vi "SVFA Compensate Phase for Ref Freq and Harm (Complex) (1 Ch).vi"(0 "complex spectrum":T7={"complex spectrum response"={"f0"=0.0, "df"=1.0, "complex spectrum"=[]}, "spectrum info"={"channel name"="", "description"="", "x-axis units"=0, "spectral info"={"spectrum type"=enum."Power [Magnitude^2]", "linear/dB"=enum."linear", "window"=0, "window size"=0, "FFT size"=0}, "engineering units"=0, "custom label"="", "dB reference [EU]"=0.0, "peak units"=enum."rms", "weighting filter"=0, "spectral density?"=FALSE, "unit label"="", "spectrum skewed?"=FALSE, "complimentary spectrum units"=enum."none"}} {"spectrum info"."x-axis units" items=["Time (s)"=0, "Frequency-CB (Hz)"=1, "Frequency-CPB (Hz)"=1248, "Frequency-Arbitrary (Hz)"=2357, "Quefrency (s)"=2, "Revolutions (rev)"=3, "Order"=4, "Speed (RPM)"=11, "Speed (rad/s)"=21, "Index"=65535]; "spectrum info"."weighting filter" items=["Linear", "A-weighting", "B-weighting", "C-weighting", "ITU-R 468-4", "Dolby", "CCITT", "C-message", "Wb", "Wc", "Wd", "We", "Wf", "Wh", "Wj", "Wk", "Wm", "AES17 20 kHz lowpass", "AES17 40 kHz lowpass", "AES17 20 kHz highpass", "AES17 40 kHz highpass"]; "spectrum info"."dB reference [EU]" format="%.2f"; "spectrum info"."engineering units" items=["custom..."=0, "V"=1, "A"=21, "C"=30, "pC"=31, "s"=32, "-"=29, "Pa"=2, "N"=20, "g"=3, "m/s^2"=4, "m/s"=5, "m"=6, "mm/s"=12, "mm"=13, "micron/s"=14, "micron"=15, "in/s^2"=7, "in/s"=8, "in"=9, "mil/s"=10, "mil"=11, "rad/s^2"=16, "rad/s"=17, "rad"=18, "deg/s^2"=26, "deg/s"=27, "deg"=28, "RPM"=22, "cycle/s^2"=23, "Hz"=24, "cycle"=25, "strain"=19]; "spectrum info"."spectral info"."window" items=["None "=0, "Hanning"=1, "Hamming"=2, "Blackman-Harris"=3, "Exact Blackman"=4, "Blackman"=5, "Flat Top"=6, "4 Term B-Harris "=7, "7 Term B-Harris"=8, "Low Sidelobe"=9, "Force - Exponential"=10, "Gaussian"=62]; "complex spectrum response"."complex spectrum" format="%.2f"; "complex spectrum response"."df" format="%.2f"; "complex spectrum response"."f0" format="%.2f"}, 2 "reference frequency [Hz]":dbl=-1.0, 3 "advanced span [Hz]":dbl, 5 "error in":errorcluster) -> (14 "phase compensated complex spectrum":T7={"complex spectrum response"={"f0"=0.0, "df"=1.0, "complex spectrum"=[]}, "spectrum info"={"channel name"="", "description"="", "x-axis units"=0, "spectral info"={"spectrum type"=enum."Power [Magnitude^2]", "linear/dB"=enum."linear", "window"=0, "window size"=0, "FFT size"=0}, "engineering units"=0, "custom label"="", "dB reference [EU]"=0.0, "peak units"=enum."rms", "weighting filter"=0, "spectral density?"=FALSE, "unit label"="", "spectrum skewed?"=FALSE, "complimentary spectrum units"=enum."none"}} {"spectrum info"."x-axis units" items=["Time (s)"=0, "Frequency-CB (Hz)"=1, "Frequency-CPB (Hz)"=1248, "Frequency-Arbitrary (Hz)"=2357, "Quefrency (s)"=2, "Revolutions (rev)"=3, "Order"=4, "Speed (RPM)"=11, "Speed (rad/s)"=21, "Index"=65535]; "spectrum info"."weighting filter" items=["Linear", "A-weighting", "B-weighting", "C-weighting", "ITU-R 468-4", "Dolby", "CCITT", "C-message", "Wb", "Wc", "Wd", "We", "Wf", "Wh", "Wj", "Wk", "Wm", "AES17 20 kHz lowpass", "AES17 40 kHz lowpass", "AES17 20 kHz highpass", "AES17 40 kHz highpass"]; "spectrum info"."dB reference [EU]" format="%.2f"; "spectrum info"."engineering units" items=["custom..."=0, "V"=1, "A"=21, "C"=30, "pC"=31, "s"=32, "-"=29, "Pa"=2, "N"=20, "g"=3, "m/s^2"=4, "m/s"=5, "m"=6, "mm/s"=12, "mm"=13, "micron/s"=14, "micron"=15, "in/s^2"=7, "in/s"=8, "in"=9, "mil/s"=10, "mil"=11, "rad/s^2"=16, "rad/s"=17, "rad"=18, "deg/s^2"=26, "deg/s"=27, "deg"=28, "RPM"=22, "cycle/s^2"=23, "Hz"=24, "cycle"=25, "strain"=19]; "spectrum info"."spectral info"."window" items=["None "=0, "Hanning"=1, "Hamming"=2, "Blackman-Harris"=3, "Exact Blackman"=4, "Blackman"=5, "Flat Top"=6, "4 Term B-Harris "=7, "7 Term B-Harris"=8, "Low Sidelobe"=9, "Force - Exponential"=10, "Gaussian"=62]; "complex spectrum response"."complex spectrum" format="%.2f"; "complex spectrum response"."df" format="%.2f"; "complex spectrum response"."f0" format="%.2f"}, 19 "error out":errorcluster)   [LabVIEW 2017]
doc: "Use this VI to enable vector averaging of complex spectra even when the frequencies of interest do not have constant phase incidence in the measurement window (analysis block)."
uses:
  <vilib>/addons/_NISVFA/_Shared subVIs/Controls/svc_Spectrum Info.ctl
  <vilib>/addons/_NISVFA/_Shared subVIs/Controls/svc_X-Axis Units.ctl
  <vilib>/addons/_NISVFA/_Shared subVIs/Controls/svc_Spectrum Type.ctl
  <vilib>/addons/_NISVFA/_Shared subVIs/Controls/svc_Engineering Units Text Ring.ctl
  <vilib>/addons/_NISVFA/_Shared subVIs/Controls/svc_Weighting Filter Text Ring.ctl
  <vilib>/addons/_NISVFA/_Shared subVIs/Controls/svc_Complimentary Spectrum Units.ctl
  <vilib>/addons/_NISVFA/_Spectrum Processing/SVFA Extract Single Tone Information (Complex) (1 Ch).vi
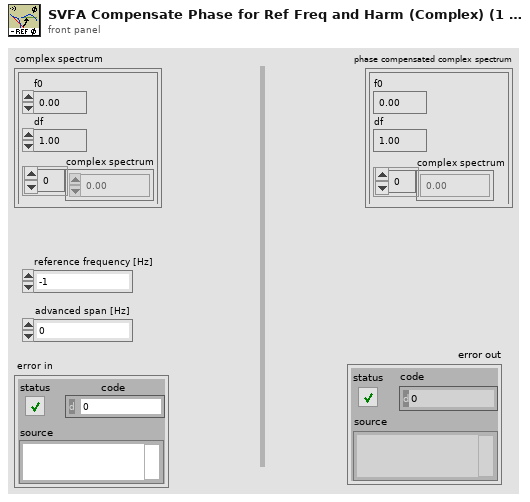
[diagram p1: front panel]
types:
  T1 = typedef "svc_Spectrum Info.ctl" = cluster{"channel name":string, "description":string, "x-axis units":T2, "spectral info":cluster{"spectrum type":T3, "linear/dB":enum16{"linear", "dB"}, "window":u16, "window size":i32, "FFT size":i32}, "engineering units":T4, "custom label":string, "dB reference [EU]":dbl, "peak units":enum16{"rms", "peak", "peak-peak"}, "weighting filter":T5, "spectral density?":bool, "unit label":string, "spectrum skewed?":bool, "complimentary spectrum units":T6}
  T2 = typedef "svc_X-Axis Units.ctl" = u16
  T3 = typedef "svc_Spectrum Type.ctl" = enum16{"FFT Spectrum [complex]", "Amplitude [Magnitude]", "Power [Magnitude^2]", "Cross Spectrum [complex]", "Frequency Response [Complex]"}
  T4 = typedef "svc_Engineering Units Text Ring.ctl" = u16
  T5 = typedef "svc_Weighting Filter Text Ring.ctl" = u16
  T6 = typedef "svc_Complimentary Spectrum Units.ctl" = enum16{"none", "radians", "degrees", "cycles", "imaginary"}
  T7 = cluster{"complex spectrum response":cluster{"f0":dbl, "df":dbl, "complex spectrum":cdb[]}, "spectrum info":T1}
  T8 = enum32{"none", "input signal", "detected signal", "residual signal"}
  T9 = cluster{"frequency [Hz]":dbl, "amplitude [EU pk]":dbl, "phase (deg)":dbl}
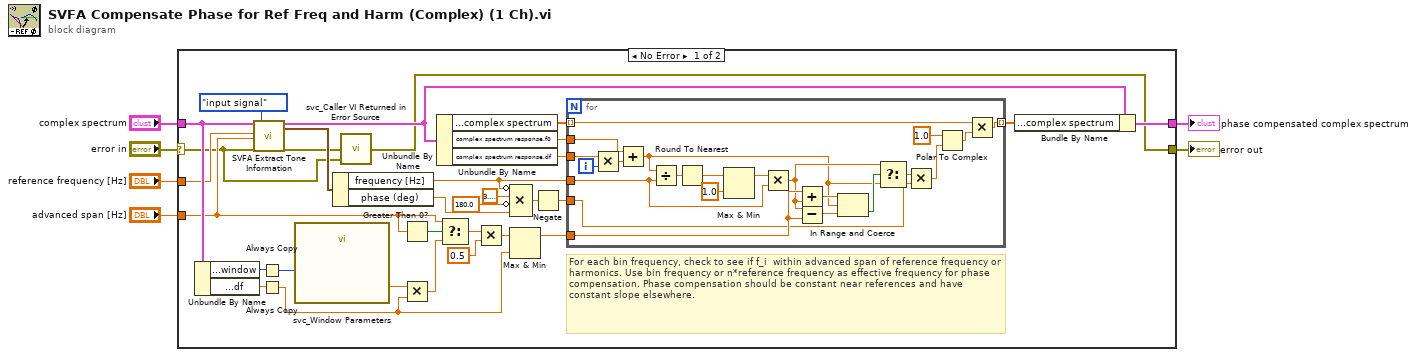
[diagram p0: block diagram]
diagram:
  n1 = case shown="No Error" "error in" {
    selector: "error in" -> [w7 w61]
    tunnel: "complex spectrum" -> [w35 w60]
    tunnel: "advanced span [Hz]" -> [w34 _]
    tunnel: "reference frequency [Hz]" -> [w33 _]
    tunnel: [w8 w61] -> w3
    tunnel: [w30 w60] -> w1
    frame No Error {
      # "For each bin frequency, check to see if f_i  within advanced span of reference frequency or harmonics. Use bin frequency or n*reference frequency as effective frequency for phase compensation. Phase compensation should be constant near references and have constant slope elsewhere."
      n2 = Unbundle By Name(w35) -> ("spectrum info.spectral info.window"=w37:u16, "complex spectrum response.df"=w32:dbl)
      n3 = call-poly <vilib>:"SVFA Extract Tone Information.vi"("complex spectrum"=w35, "expected frequency [Hz]"=w33, "advanced span [Hz]"=w34, "error in"=w7, "export signals"=T8."input signal") -> ("complex spectrum"=w17:T7, "detected tone"=w25:T9, "error out"=w9:errorcluster)  [unwired: 11 in, 1 out]
      n4 = Always Copy(1:w37) -> (0:w36:u16)
      n5 = Always Copy(1:w32) -> (0:w31:dbl)
      n6 = call <vilib>:"svc_Window Parameters.vi"("window"=w36) -> ("maximum BW"=w28:dbl)  [unwired: 7 in, 3 out]
      n7 = Unbundle By Name(w25) -> ("frequency [Hz]"=w11:dbl, "phase (deg)"=w13:dbl)
      n8 = call <vilib>:"svc_Caller VI Returned in Error Source.vi"("warning input to caller"=w7, "error in (no error)"=w9) -> ("error out"=w8:errorcluster)  [unwired: 3 in]
      n9 = Greater Than 0?(x=w34) -> (x > 0?=w29:bool)
      n10 = Multiply(x=w28, y=w31) -> (x*y=w27:dbl)
      n11 = Unbundle By Name(w17) -> ("complex spectrum response.complex spectrum"=w22:cdb[], "complex spectrum response.f0"=w21:dbl, "complex spectrum response.df"=w20:dbl)
      n12 = Select(t=w34, s=w29, f=w27) -> (s? t:f=w24:dbl)
      n13 = Multiply(x=w24, y=0.5 ("value")) -> (x*y=w23:dbl)
      n14 = Compound Arithmetic op=MULTIPLY(invert w11, 3.141592653589793 ("x"), invert 180.0 ("y"), w13) -> (w12:dbl)
      n15 = Max & Min(x=w23, y=w31) -> (max(x,y)=w19:dbl)  [unwired: 1 out]
      n16 = Negate(x=w12) -> (-x=w10:dbl)
      n17 = for {
        tunnel: w21 -> [w56]
        tunnel: w20 -> [w59]
        tunnel: w10 -> [w42]
        tunnel: w19 -> [w51]
        tunnel: w22 -> [w44] mode=indexing
        tunnel: [w43] -> w18 mode=indexing
        tunnel: w11 -> [w38]
        i -> [w58]
        n18 = Multiply(x=w59, y=w58) -> (x*y=w57:dbl)
        n19 = Add(x=w56, y=w57) -> (x+y=w45:dbl)
        n20 = Divide(x=w45, y=w38) -> (x/y=w55:dbl)
        n21 = Round To Nearest(number=w55) -> (nearest integer value=w41:dbl)
        n22 = Max & Min(x=w41, y=1.0 ("x")) -> (max(x,y)=w40:dbl)  [unwired: 1 out]
        n23 = Multiply(x=w40, y=w38) -> (x*y=w50:dbl)
        n24 = Add(x=w51, y=w50) -> (x+y=w54:dbl)
        n25 = Subtract(x=w50, y=w51) -> (x-y=w53:dbl)
        n26 = In Range and Coerce(upper limit=w54, x=w45, lower limit=w53) -> (In Range?=w52:bool)  [unwired: 1 out]
        n27 = Select(t=w50, s=w52, f=w45) -> (s? t:f=w49:dbl)
        n28 = Multiply(x=w49, y=w42) -> (x*y=w46:dbl)
        n29 = Polar To Complex(1:w46, 2:1.0 ("x")) -> (0:w47:cdb)
        n30 = Multiply(x=w44, y=w47) -> (x*y=w43:cdb)
      }
      n31 = Bundle By Name(cluster=w17, "complex spectrum response.complex spectrum"=w18) -> (w30:T7)
    }
    frame Error {
    }
  }
  "phase compensated complex spectrum" <- w1
  "error out" <- w3
